vi "VI AK Master Amium.vi"(8 "error in (no error)":errorcluster caption="Fehler (Eingang, kein Fehler)") -> (0 "error out":errorcluster)   [LabVIEW 2020, in "Amium PNS.lvlib" / "AK Kommunikation.lvlib"]
uses:
  AK Kommunikation.lvlib
  Aktionen AK Amium.ctl
  Allgemein/Zykluszeiterfassung Aktionen.ctl
  Seiten/FT-IR/AK interface/Aktionen AK.ctl
  TCP Timeout Aktionen - Amium.ctl
  Aktion FGV Amium Daten.ctl
  Temperaturregler Cluster.ctl
  Stoerungen/Stoerungen Messgeraet/Aktionen Kommunikation Stoerung.ctl
  Seiten/FT-IR/AK interface/AK-Interface.lvlib
  Allgemein/allgemeine Sub-VIs.lvlib
  Stoerungen/Stoerungen.lvlib
  Amium PNS.lvlib
panel:
  out "Hz":sgl=80.0 format="%#.1f"
  out "Zustand":T1
  out "initialisieren":errorcluster caption="initiálisieren"
  out "Diagramm":u32(graph)
  out "AK Komm":errorcluster
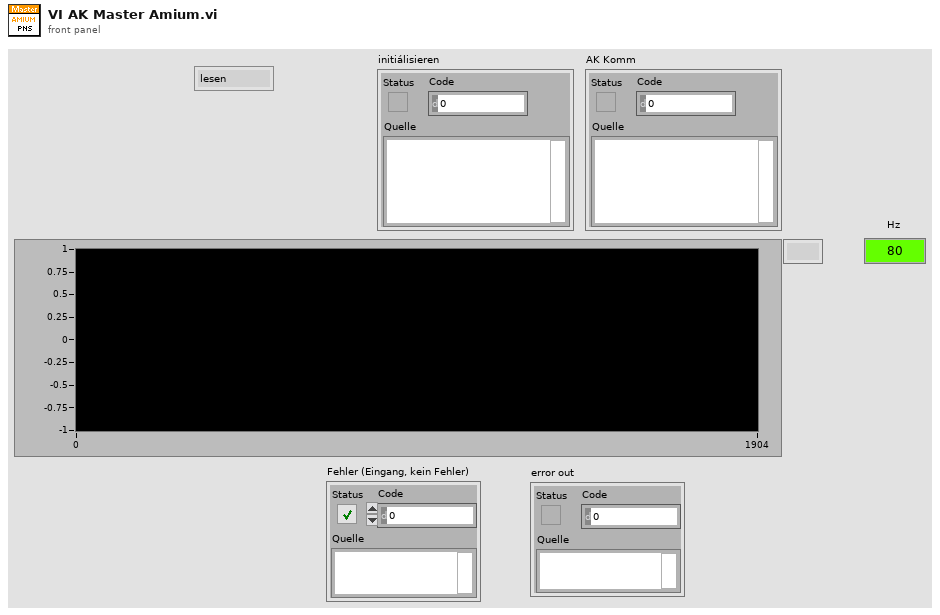
[diagram p1: front panel]
types:
  T1 = typedef "Amium PNS.lvlib/AK Kommunikation.lvlib/Aktionen AK Amium.ctl" = enum16{"lesen", "initialisieren", "beenden", "AK Komm"}
  T2 = typedef "Amium PNS.lvlib/Temperaturregler Cluster.ctl" = cluster{"Istwert":sgl, "Sollwert":sgl, "Stellgröße":sgl, "Status":sgl, "Error":sgl}
  T3 = typedef "Amium PNS.lvlib/Aktion FGV Amium Daten.ctl" = enum16{"lesen", "Komm Daten", "Daten", "Error", "Regler", "Grenzwerte", "laden", "speichern"}
  T4 = typedef "Amium PNS.lvlib/AK Kommunikation.lvlib/TCP Timeout Aktionen - Amium.ctl" = enum16{"lesen", "setzen"}
  T5 = typedef "FT-IR.lvlib/AK-Interface.lvlib/Aktionen AK.ctl" = enum16{"lesen", "initialisieren", "beenden", "AK Komm"}
  T6 = typedef "allgemeine Sub-VIs.lvlib/Zykluszeiterfassung Aktionen.ctl" = enum16{"lesen", "init", "Messdaten1", "ToolWeb", "AK FT-IR", "AK Extern", "AK Amium"}
  T7 = typedef "Stoerungen.lvlib/Aktionen Kommunikation Stoerung.ctl" = enum16{"lesen", "init", "FT-IR Komm", "FT-IR Betriebsart", "FT-IR Hintergrund", "cRIO Komm", "PNS Komm", "Dichtheitstest", "Life Bit", "FTIR Komm AK", "PMA Komm", "FID Komm", "PMA Cal", "FID Ch4 Cal", "FID THC Cal", "Cal Timeout", "VFS 1 Komm", "VFS 2 Komm", "VFS 3 Komm", "VFS 4 Komm", "TRE 08 Komm", "CG-Test vorzeitig", "CG-Test Span 1", "CG-Test Span 2", "CG-Test Span 3", "CG-Test Messgas", "CG-Test löschen", "Test", "Amium AK", "AK Recept konfig", "AK Name konfig", "AK EKFG konfig"}
  T8 = typedef "Amium PNS.lvlib/Kommunikation Daten Cluster.ctl" = cluster{"IP Adresse":string, "Port":i16}
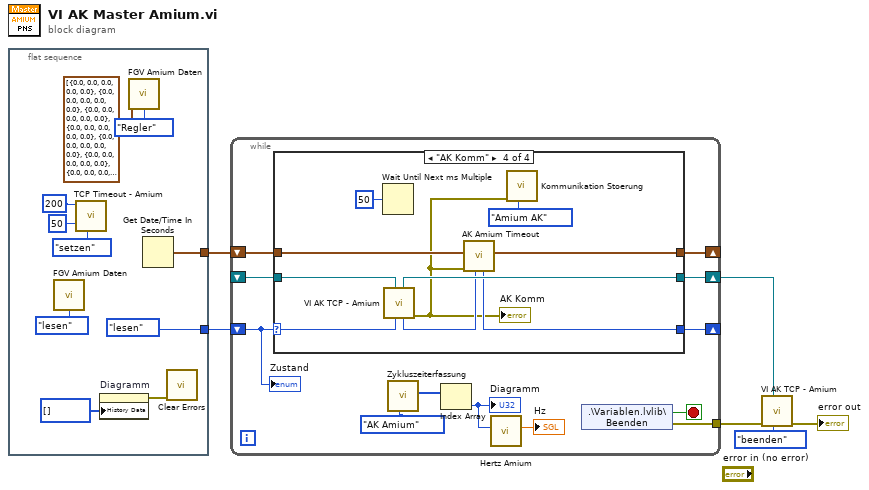
[diagram p0: block diagram]
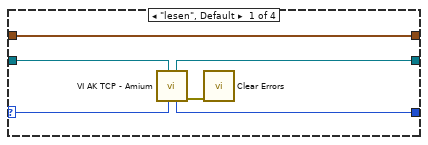
[diagram p2: hidden frame]
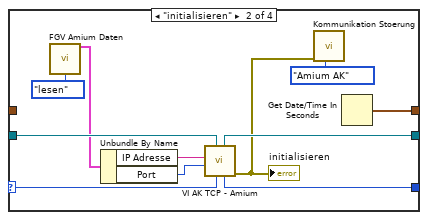
[diagram p3: hidden frame]
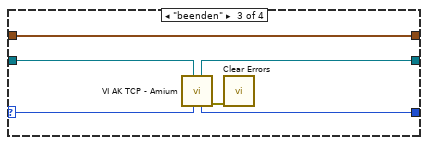
[diagram p4: hidden frame]
diagram:
  n1 = flat-sequence {
    tunnel: [Aktionen_AK."lesen" ("Aktionen")] -> w3
    tunnel: [w16] -> w5
    frame #0 {
      n2 = call "FGV Amium Daten.vi"("Aktion"=Aktion_FGV_Amium_Daten."lesen") -> ()  [unwired: 9 in, 6 out]
      n3 = call "TCP Timeout - Amium.vi"("Aktionen Timeout"=TCP_Timeout_Aktionen_-_Amium."setzen", "Timeout lesen"=50, "Timeout schreiben"=200) -> ()  [unwired: 7 in, 2 out]
      n4 = property on="Diagramm" class="SVDiagr (strikt)"("History Data"=u32[] [] ("Historiendaten")) -> (error out=w14:errorcluster)  [unwired: 2 in, 1 out]
      n5 = call "FGV Amium Daten.vi"("Regler"=T2[] [{"Istwert"=0.0, "Sollwert"=0.0, "Stellgröße"=0.0, "Status"=0.0, "Error"=0.0}, {"Istwert"=0.0, "Sollwert"=0.0, "Stellgröße"=0.0, "Status"=0.0, "Error"=0.0}, {"Istwert"=0.0, "Sollwert"=0.0, "Stellgröße"=0.0, "Status"=0.0, "Error"=0.0}, {"Istwert"=0.0, "Sollwert"=0.0, "Stellgröße"=0.0, "Status"=0.0, "Error"=0.0}, {"Istwert"=0.0, "Sollwert"=0.0, "Stellgröße"=0.0, "Status"=0.0, "Error"=0.0}, {"Istwert"=0.0, "Sollwert"=0.0, "Stellgröße"=0.0, "Status"=0.0, "Error"=0.0}, {"Istwert"=0.0, "Sollwert"=0.0, "Stellgröße"=0.0, "Status"=0.0, "Error"=0.0}, {"Istwert"=0.0, "Sollwert"=0.0, "Stellgröße"=0.0, "Status"=0.0, "Error"=0.0}, {"Istwert"=0.0, "Sollwert"=0.0, "Stellgröße"=0.0, "Status"=0.0, "Error"=0.0}, {"Istwert"=0.0, "Sollwert"=0.0, "Stellgröße"=0.0, "Status"=0.0, "Error"=0.0}, {"Istwert"=0.0, "Sollwert"=0.0, "Stellgröße"=0.0, "Status"=0.0, "Error"=0.0}, {"Istwert"=0.0, "Sollwert"=0.0, "Stellgröße"=0.0, "Status"=0.0, "Error"=0.0}, {"Istwert"=0.0, "Sollwert"=0.0, "Stellgröße"=0.0, "Status"=0.0, "Error"=0.0}, {"Istwert"=0.0, "Sollwert"=0.0, "Stellgröße"=0.0, "Status"=0.0, "Error"=0.0}, {"Istwert"=0.0, "Sollwert"=0.0, "Stellgröße"=0.0, "Status"=0.0, "Error"=0.0}, {"Istwert"=0.0, "Sollwert"=0.0, "Stellgröße"=0.0, "Status"=0.0, "Error"=0.0}, {"Istwert"=0.0, "Sollwert"=0.0, "Stellgröße"=0.0, "Status"=0.0, "Error"=0.0}, {"Istwert"=0.0, "Sollwert"=0.0, "Stellgröße"=0.0, "Status"=0.0, "Error"=0.0}, {"Istwert"=0.0, "Sollwert"=0.0, "Stellgröße"=0.0, "Status"=0.0, "Error"=0.0}, {"Istwert"=0.0, "Sollwert"=0.0, "Stellgröße"=0.0, "Status"=0.0, "Error"=0.0}, {"Istwert"=0.0, "Sollwert"=0.0, "Stellgröße"=0.0, "Status"=0.0, "Error"=0.0}], "Aktion"=Aktion_FGV_Amium_Daten."Regler") -> ()  [unwired: 8 in, 6 out]
      n6 = Get Date/Time In Seconds() -> (seconds since 1Jan1904=w16:timestamp)
      n7 = call <vilib>:"Clear Errors.vi"("error in (no error)"=w14) -> ()  [unwired: 5 in, 2 out]
    }
  }
  n8 = while {
    shift-right: [w27] -> _
    shift-left: w3 -> [w28]
    shift-right: [w26] -> _
    shift-left: w5 -> [w25]
    tunnel: [w24] -> w6
    shift-right: [w22] -> w4
    shift-left: _ -> [w21]
    stop <- w23 stop-if-true
    n9 = case shown="\"AK Komm\"" w28 {
      selector: w28 -> [w33 w45 w51 w58]
      tunnel: [w29 w41 w46 w57] -> w27
      tunnel: [w34 w44 w50 w56] -> w26
      tunnel: w25 -> [w34 _ w50 w61]
      tunnel: [w30 w42 w47 w60] -> w22
      tunnel: w21 -> [w31 w43 w48 w59]
      frame "lesen", Default {
        n10 = call "VI AK TCP - Amium.vi"("Aktionen"=w33, "connection ID"=w31) -> ("error out"=w32:errorcluster, "Aktionen"=w29:T1, "connection ID"=w30:refnum<k5>)  [unwired: 6 in, 1 out]
        n11 = call <vilib>:"Clear Errors.vi"("error in (no error)"=w32) -> ()  [unwired: 5 in, 2 out]
      }
      frame "initialisieren" {
        n12 = call "FGV Amium Daten.vi"("Aktion"=Aktion_FGV_Amium_Daten."lesen") -> ("Amium Komm Daten"=w37:T8)  [unwired: 9 in, 5 out]
        n13 = Unbundle By Name(w37) -> ("IP Adresse"=w36:string, "Port"=w35:i16)
        n14 = call "VI AK TCP - Amium.vi"("Aktionen"=w45, "connection ID"=w43, "Port"=w35, "IP-Adresse:"=w36) -> ("error out"=w39:errorcluster, "Aktionen"=w41:T1, "connection ID"=w42:refnum<k5>)  [unwired: 4 in, 1 out]
        "initialisieren" <- w39
        n15 = call "Kommunikation Stoerung.vi"("Aktionen"=Aktionen_Kommunikation_Stoerung."Amium AK", "error in"=w39) -> ()  [unwired: 9 in, 1 out]
        n16 = Get Date/Time In Seconds() -> (seconds since 1Jan1904=w44:timestamp)
      }
      frame "beenden" {
        n17 = call "VI AK TCP - Amium.vi"("Aktionen"=w51, "connection ID"=w48) -> ("error out"=w49:errorcluster, "Aktionen"=w46:T1, "connection ID"=w47:refnum<k5>)  [unwired: 6 in, 1 out]
        n18 = call <vilib>:"Clear Errors.vi"("error in (no error)"=w49) -> ()  [unwired: 5 in, 2 out]
      }
      frame "AK Komm" {
        n19 = Wait Until Next ms Multiple(millisecond multiple=u32 50 ("ms")) -> ()  [unwired: 1 out]
        n20 = call "VI AK TCP - Amium.vi"("Aktionen"=w58, "connection ID"=w59) -> ("error out"=w54:errorcluster, "Aktionen"=w55:T1, "connection ID"=w60:refnum<k5>)  [unwired: 6 in, 1 out]
        "AK Komm" <- w54
        n21 = call "AK Amium Timeout.vi"("Aktionen"=w55, "Fehler"=w54, "Zeitstempel"=w61) -> ("Zeitstempel"=w56:timestamp, "Aktionen"=w57:T1)  [unwired: 7 in]
        n22 = call "Kommunikation Stoerung.vi"("Aktionen"=Aktionen_Kommunikation_Stoerung."Amium AK", "error in"=w54) -> ()  [unwired: 9 in, 1 out]
      }
    }
    n23 = call "Zykluszeiterfassung.vi"("Aktionen"=Zykluszeiterfassung_Aktionen."AK Amium") -> ("Zykluszeiten"=w19:u32[])  [unwired: 10 in]
    n24 = Index Array(array=w19) -> (element=w18:u32)  [unwired: 1 in]
    "Diagramm" <- w18
    n25 = call "Hertz Amium.vi"("Zeit [ms]"=w18) -> ("Hertz"=→"Hz":sgl)  [unwired: 10 in]
    n26 = shared-variable ".\\Variablen.lvlib\\Beenden"() -> (w23:bool, error out=w24:errorcluster)  [unwired: 1 in]
    "Zustand" <- w28
  }
  n27 = call "VI AK TCP - Amium.vi"("Aktionen"=Aktionen_AK_Amium."beenden", "connection ID"=w4, "error in"=w6) -> ("error out"=→"error out":errorcluster)  [unwired: 5 in, 3 out]
